vi "VarArray_Delete elements.vi"(8 "Error In":errorcluster, 9 "Index Array In":i32[](array[numeric]), 11 "Array In":variant[](array[variant])) -> (0 "Error Out":errorcluster, 1 "Deleted Elements Out":variant[](array[variant]), 3 "Array Out":variant[](array[variant]))   [LabVIEW 2015]
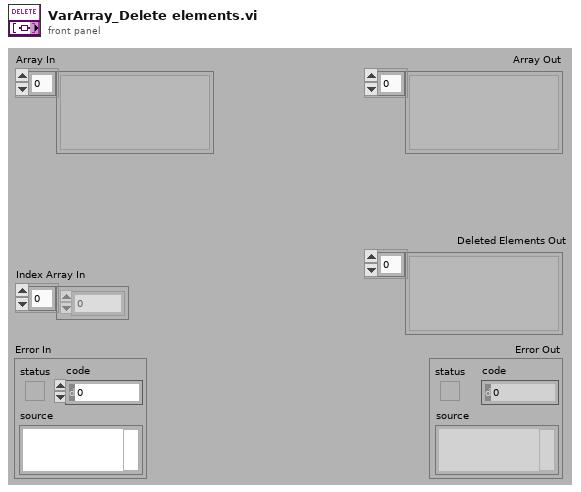
[diagram p1: front panel]
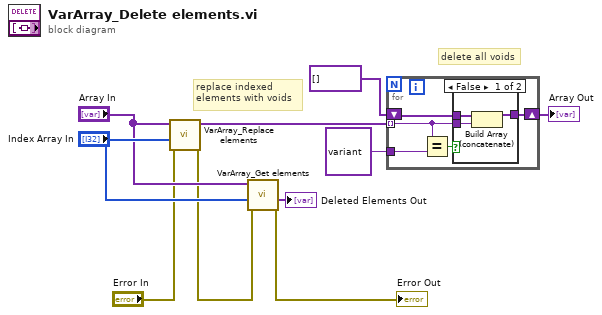
[diagram p0: block diagram]
diagram:
  # "delete all voids"
  # "replace indexed\nelements with voids"
  n1 = call "VarArray_Replace elements.vi"("Error In"="Error In", "Index Array In"="Index Array In", "Array In In In"="Array In") -> ("Error Out"=w2:errorcluster, "Array Out"=w7:variant[])  [unwired: 5 in, 2 out]
  n2 = call "VarArray_Get elements.vi"("Error In"=w2, "Index Array In"="Index Array In", "Array In In"="Array In") -> ("Error Out"=→"Error Out":errorcluster, "Selected Array Out"=→"Deleted Elements Out":variant[])  [unwired: 7 in]
  n3 = for {
    shift-right: [w12] -> w6
    shift-left: variant[] [] -> [w11]
    tunnel: w7 -> [w13] mode=indexing
    tunnel: variant ("Variant") -> [w15]
    n4 = Equal?(x=w13, y=w15) -> (x = y?=w14:bool)
    n5 = case shown="False" w14 {
      tunnel: w13 -> [w18 _]
      tunnel: [w17 w19] -> w12
      tunnel: w11 -> [w16 w19]
      frame False {
        n6 = Build Array (concatenate)(w16, w18) -> (w17:variant[])
      }
      frame True {
      }
    }
  }
  "Array Out" <- w6
